vi "FlatToRichcif_waveformmonitor_Empty.vi"(5 "OutputClusterType":T1, 11 "InputCluster":T2) -> (3 "OutputCluster":T1)   [LabVIEW 2021, in "CIFWaveformMonitor_server.lvlib"]
uses:
  cif_waveformmonitor_Empty_Flat.ctl
  cif_waveformmonitor_Empty.ctl
  CIFWaveformMonitor_server.lvlib
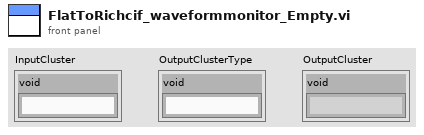
[diagram p1: front panel]
types:
  T1 = typedef "CIFWaveformMonitor_server.lvlib/cif_waveformmonitor_Empty.ctl" = cluster{"void":string}
  T2 = typedef "CIFWaveformMonitor_server.lvlib/cif_waveformmonitor_Empty_Flat.ctl" = cluster{"void":string}
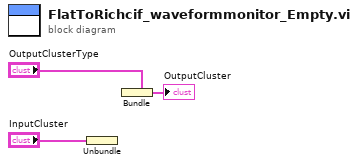
[diagram p0: block diagram]
diagram:
  n1 = Unbundle "Unbundle"("InputCluster") -> ()  [unwired: 1 out]
  n2 = Bundle "Bundle"(cluster="OutputClusterType") -> (→"OutputCluster":T1)  [unwired: 1 in]
